vi "ActionVIOnCompile.vi"(8 "error in (no error)":errorcluster, 11 "Device Item Ref in":T1 format="%.0x") -> (0 "error out":errorcluster)   [LabVIEW 2023, in "Vires VTD System Explorer.lvlib"]
uses:
  Vires VTD System Explorer.lvlib
  <vilib>/NI VeriStand/Custom Device API/Custom Device Item Ref.ctl
  Shared/Compiled.Settings.ctl
  RDB Data.ctl
  RDB/RDB Object.ctl
  RDB/RDB Player Object.ctl
  Shared/Network Settings.ctl
  Shared/Protocol.ctl
  Shared/SensorInfos.ctl
  Shared/SensorInfo.ctl
  Shared/Sensor Name.ctl
  MM/MM Data.ctl
  MM/MM Objects.ctl
  MM/MM Object.ctl
  Shared/Timedloop Settings.ctl
  Shared/Constants.vi
  <vilib>/NI VeriStand/Custom Device Tools/Custom Device Utility Library/NI VeriStand - Search for Item by Name.vi
  <vilib>/NI VeriStand/Custom Device API/Get Item Property (Variant).vi
  <vilib>/NI VeriStand/Custom Device API/Set Item Property (Variant).vi
  <vilib>/NI VeriStand/Custom Device API/Custom Device API.lvlib
  <vilib>/NI VeriStand/Custom Device Tools/Custom Device Utility Library/Custom Device Utility Library.lvlib
  <vilib>/NI/NIVS Inline Async API/_Data Access System Explorer/Data Access System Explorer.lvlib
  Shared/Vires VTD Shared.lvlib
  RDB/RDB.lvlib
  MM/MM.lvlib
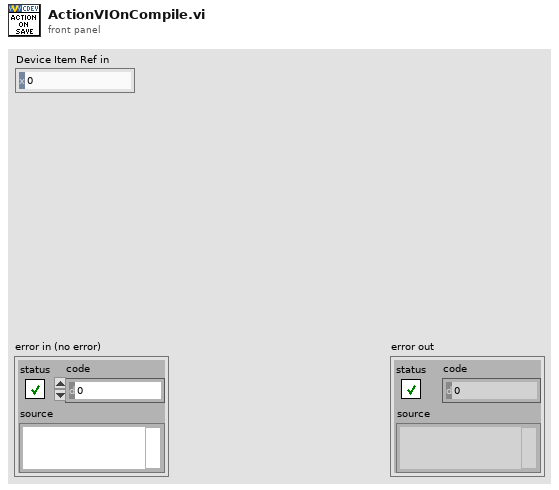
[diagram p1: front panel]
types:
  T1 = typedef "Custom Device API.lvlib/Custom Device Item Ref.ctl" = u64
  T2 = cluster{"Name":string, "Type":enum16{"Output/Write", "Input/Read", "Input/ReadWrite"}, "VS Refs":T1[]}
  T3 = enum16{"Output/Write", "Input/Read", "Input/ReadWrite"}
  T4 = typedef "Vires VTD Shared.lvlib/Compiled.Settings.ctl" = cluster{"Name":string, "RDB Data Receive ":T5, "RDB Data Sent":T5, "vclient":path, "Network Settings":T8, "SensorInfos":T10, "mmanager":path, "Scenario Paths":string[], "Custom SCP Commands":string[], "Timed Loop Settings for TaskControl":T16, "Timed Loop Settings for ModuleManager":T16}
  T5 = typedef "Vires VTD Shared.lvlib/RDB Data.ctl" = T6[]
  T6 = typedef "RDB.lvlib/RDB Object.ctl" = cluster{"pkID":i32, "RDB Player Objects":T7[]}
  T7 = typedef "RDB.lvlib/RDB Player Object.ctl" = cluster{"PlayerID":i32, "Signals":string[], "adv para":i32}
  T8 = typedef "Vires VTD Shared.lvlib/Network Settings.ctl" = cluster{"IP adress":string, "RDB":cluster{"Protocol":T9, "Tx Port":u16, "Rx Port":u16, "Buffer Size":i32, "Timeout":u16}, "SCP":cluster{"Protocol":T9, "Tx Port":u16, "Rx Port":u16, "Buffer Size":i32, "Timeout":u16}}
  T9 = typedef "Vires VTD Shared.lvlib/Protocol.ctl" = enum16{"UDP", "TCP"}
  T10 = typedef "Vires VTD Shared.lvlib/SensorInfos.ctl" = T11[]
  T11 = typedef "Vires VTD Shared.lvlib/SensorInfo.ctl" = cluster{"Sensor Name":T12, "Protocol":T9, "Network port":i32, "# Culled Objects":i32, "PlayerID":u8, "MM Data":T13}
  T12 = typedef "Vires VTD Shared.lvlib/Sensor Name.ctl" = string
  T13 = typedef "Vires VTD Shared.lvlib/MM Data.ctl" = T14[]
  T14 = typedef "MM.lvlib/MM Objects.ctl" = cluster{"pkID":i32, "MM Objects":T15[]}
  T15 = typedef "MM.lvlib/MM Object.ctl" = cluster{"Object":i32, "Signals":string[]}
  T16 = typedef "Vires VTD Shared.lvlib/Timedloop Settings.ctl" = cluster{"Period(ms)":i64, "Priority":i32, "Processor":i32}
  T17 = typedef "Custom Device API.lvlib/Custom Device Item Info.ctl" = cluster{"Name":string, "Is Channel":bool, "GUID":string, "Is Waveform":bool}
  T18 = cluster{"Name":string, "Type":enum16{"Output/Write", "Input/Read", "Input/ReadWrite"}, "VS Refs":T1[]}[]
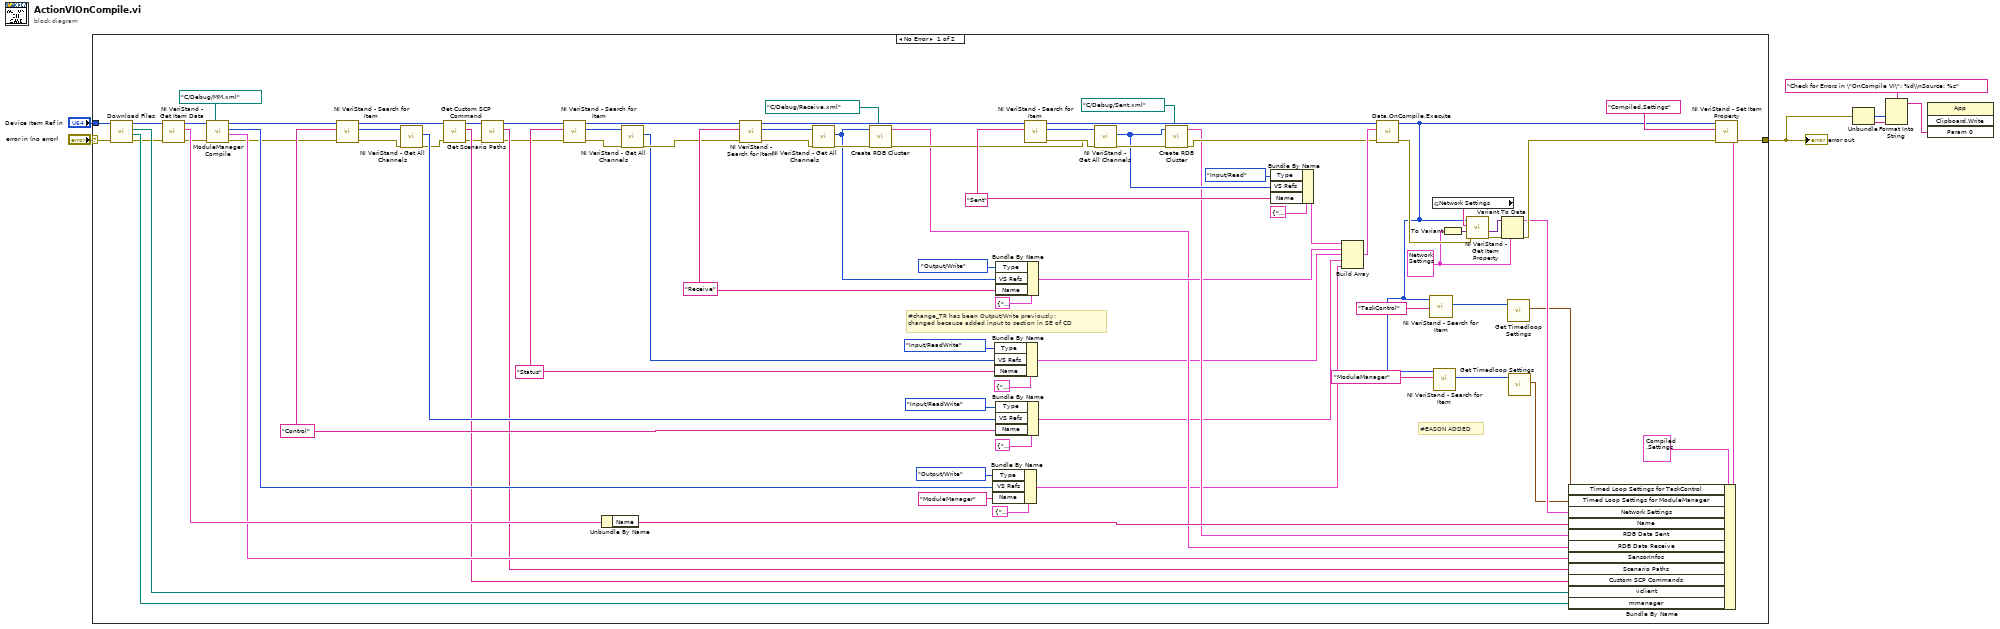
[diagram p0: block diagram]
diagram:
  n1 = case shown="No Error" "error in (no error)" {
    selector: "error in (no error)" -> [w64 w95]
    tunnel: [w66 w95] -> w3
    tunnel: "Device Item Ref in" -> [w65 _]
    frame No Error {
      w30 = "Control" ("Item Name")
      w51 = "Status" ("Item Name")
      w40 = T8 {"IP adress"="127.0.0.1", "RDB"={"Protocol"=enum."UDP", "Tx Port"=48190, "Rx Port"=8192, "Buffer Size"=48190, "Timeout"=10}, "SCP"={"Protocol"=enum."UDP", "Tx Port"=48190, "Rx Port"=8192, "Buffer Size"=48190, "Timeout"=10}} ("UDP Settings")
      w89 = "Sent" ("Item Name")
      w90 = "Receive" ("Item Name")
      # "#EASON ADDED"
      # "#change_TR has been Output/Write previously;\nchanged because added input to section in SE of CD"
      n2 = call "Download Files.vi"("error in (no error)"=w64, "Item Ref in"=w65) -> ("error out"=w20:errorcluster, "mmanager"=w41:path, "vclient"=w43:path, "Device Ref out"=w63:T1)  [unwired: 6 in]
      n3 = call <vilib>:"NI VeriStand - Get Item Data.vi"("error in (no error)"=w20, "Item Ref in"=w63) -> ("error out"=w48:errorcluster, "Item Info"=w92:T17, "Item Ref out"=w49:T1)  [unwired: 6 in, 1 out]
      n4 = call "ModuleManager Compile.vi"("datalog path"=path "C:/Debug/MM.xml", "error in"=w48, "Section Ref in"=w49) -> ("error out"=w28:errorcluster, "SensorInfos"=w42:T10, "Channel Refs"=w45:T1[], "Section Ref out"=w31:T1)  [unwired: 5 in]
      n5 = call-poly <vilib>:"NI VeriStand - Search for Item.vi"("error in"=w28, "Item Name"=w30, "Section Ref in"=w31) -> ("error out"=w33:errorcluster, "Item Ref"=w32:T1, "Section Ref out"=w24:T1)  [unwired: 5 in, 1 out]
      n6 = call <vilib>:"NI VeriStand - Get All Channels.vi"("error in"=w33, "Section Ref in"=w32) -> ("error out"=w27:errorcluster, "Channel Refs"=w29:T1[])  [unwired: 6 in, 2 out]
      n7 = call "Get Custom SCP Command.vi"("error in (no error)"=w27, "Section Ref in"=w24) -> ("error out"=w18:errorcluster, "Custom SCP Commands (str)"=w22:string[], "Section Ref out"=w23:T1)  [unwired: 7 in]
      n8 = call "Get Scenario Paths.vi"("error in (no error)"=w18, "Section Ref in"=w23) -> ("error out"=w19:errorcluster, "Scenario Paths (str)"=w21:string[], "Section Ref out"=w26:T1)  [unwired: 6 in, 1 out]
      n9 = call-poly <vilib>:"NI VeriStand - Search for Item.vi"("error in"=w19, "Item Name"=w51, "Section Ref in"=w26) -> ("error out"=w57:errorcluster, "Item Ref"=w58:T1, "Section Ref out"=w56:T1)  [unwired: 5 in, 1 out]
      n10 = Unbundle By Name(w92) -> ("Name"=w91:string)
      n11 = call <vilib>:"NI VeriStand - Get All Channels.vi"("error in"=w57, "Section Ref in"=w58) -> ("error out"=w55:errorcluster, "Channel Refs"=w52:T1[])  [unwired: 6 in, 2 out]
      n12 = call-poly <vilib>:"NI VeriStand - Search for Item.vi"("error in"=w55, "Item Name"=w90, "Section Ref in"=w56) -> ("error out"=w79:errorcluster, "Item Ref"=w78:T1, "Section Ref out"=w81:T1)  [unwired: 5 in, 1 out]
      n13 = call <vilib>:"NI VeriStand - Get All Channels.vi"("error in"=w79, "Section Ref in"=w78) -> ("error out"=w75:errorcluster, "Channel Refs"=w74:T1[])  [unwired: 6 in, 2 out]
      n14 = call "Create RDB Cluster.vi"("datalog path"=path "C:/Debug/Receive.xml", "error out"=w75, "Channel Refs"=w74) -> ("error out"=w73:errorcluster, "RDB Object"=w67:T5)  [unwired: 7 in]
      n15 = Bundle By Name(cluster=T2 {"Name"="", "Type"=enum."Output/Write", "VS Refs"=[]} ("Group"), "Type"=T3."Output/Write", "VS Refs"=w45, "Name"="ModuleManager") -> (w37:T2)
      n16 = Bundle By Name(cluster=T2 {"Name"="", "Type"=enum."Output/Write", "VS Refs"=[]} ("Group"), "Type"=T3."Input/ReadWrite", "VS Refs"=w52, "Name"=w51) -> (w50:T2)
      n17 = Bundle By Name(cluster=T2 {"Name"="", "Type"=enum."Output/Write", "VS Refs"=[]} ("Group"), "Type"=T3."Output/Write", "VS Refs"=w74, "Name"=w90) -> (w68:T2)
      n18 = Bundle By Name(cluster=T2 {"Name"="", "Type"=enum."Output/Write", "VS Refs"=[]} ("Group"), "Type"=T3."Input/ReadWrite", "VS Refs"=w29, "Name"=w30) -> (w34:T2)
      n19 = call-poly <vilib>:"NI VeriStand - Search for Item.vi"("error in"=w73, "Item Name"=w89, "Section Ref in"=w81) -> ("error out"=w77:errorcluster, "Item Ref"=w76:T1, "Section Ref out"=w82:T1)  [unwired: 5 in, 1 out]
      n20 = call <vilib>:"NI VeriStand - Get All Channels.vi"("error in"=w77, "Section Ref in"=w76) -> ("error out"=w72:errorcluster, "Channel Refs"=w71:T1[])  [unwired: 6 in, 2 out]
      n21 = call "Create RDB Cluster.vi"("datalog path"=path "C:/Debug/Sent.xml", "error out"=w72, "Channel Refs"=w71) -> ("error out"=w70:errorcluster, "RDB Object"=w69:T5)  [unwired: 7 in]
      n22 = Bundle By Name(cluster=T2 {"Name"="", "Type"=enum."Output/Write", "VS Refs"=[]} ("Group"), "Type"=T3."Input/Read", "VS Refs"=w71, "Name"=w89) -> (w87:T2)
      n23 = Build Array(w87, w68, w50, w34, w37) -> (w85:T18)
      n24 = call <vilib>:"Data.OnCompile.Execute.vi"("error in"=w70, "VS Ref Groups"=w85, "Custom Device Ref"=w82) -> ("error out"=w59:errorcluster, "Custom Device Ref"=w17:T1)  [unwired: 7 in]
      n25 = call-poly <vilib>:"NI VeriStand - Search for Item.vi"("Item Name"="TaskControl", "Section Ref in"=w17) -> ("Item Ref"=w16:T1)  [unwired: 6 in, 3 out]
      n26 = global read "Constants.vi" "Network Settings"() -> (w62:string)
      n27 = call-poly <vilib>:"NI VeriStand - Search for Item.vi"("Item Name"="ModuleManager", "Section Ref in"=w17) -> ("Item Ref"=w15:T1)  [unwired: 6 in, 3 out]
      n28 = To Variant(anything=w40) -> (Variant=w39:variant)
      n29 = call-poly <vilib>:"NI VeriStand - Get Item Property.vi"("error in (no error)"=w59, "Default Value"=w39, "Property Name"=w62, "Item Ref in"=w17) -> ("error out"=w61:errorcluster, "Value"=w60:variant)  [unwired: 4 in, 2 out]
      n30 = Variant To Data(error in=w61, type=w40, Variant=w60) -> (data=w25:T8, error out=w38:errorcluster)
      n31 = call "Get Timedloop Settings.vi"("Item Ref in"=w16) -> ("Timed Loop Settings"=w11:T16)  [unwired: 8 in, 2 out]
      n32 = call "Get Timedloop Settings.vi"("Item Ref in"=w15) -> ("Timed Loop Settings"=w12:T16)  [unwired: 8 in, 2 out]
      n33 = Bundle By Name(cluster=T4 {"Name"="", "RDB Data Receive "=[], "RDB Data Sent"=[], "vclient"=path "", "Network Settings"={"IP adress"="127.0.0.1", "RDB"={"Protocol"=enum."UDP", "Tx Port"=48190, "Rx Port"=10, "Buffer Size"=204800, "Timeout"=10}, "SCP"={"Protocol"=enum."TCP", "Tx Port"=48191, "Rx Port"=48191, "Buffer Size"=204800, "Timeout"=10}}, "SensorInfos"=[], "mmanager"=path "", "Scenario Paths"=[], "Custom SCP Commands"=[], "Timed Loop Settings for TaskControl"={"Period(ms)"=2, "Priority"=100, "Processor"=-2}, "Timed Loop Settings for ModuleManager"={"Period(ms)"=2, "Priority"=100, "Processor"=-2}} ("Compiled.Settings"), "Timed Loop Settings for TaskControl"=w11, "Timed Loop Settings for ModuleManager"=w12, "Network Settings"=w25, "Name"=w91, "RDB Data Sent"=w69, "RDB Data Receive"=w67, "SensorInfos"=w42, "Scenario Paths"=w21, "Custom SCP Commands"=w22, "vclient"=w43, "mmanager"=w41) -> (w93:T4)
      n34 = call-poly <vilib>:"NI VeriStand - Set Item Property.vi"("error in (no error)"=w38, "Value"=w93, "Property Name"="Compiled.Settings", "Item Ref in"=w17) -> ("error out"=w66:errorcluster)  [unwired: 5 in, 2 out]
    }
    frame Error {
    }
  }
  "error out" <- w3
  n35 = Unbundle(w3) -> ("code"=w4:i32, "source"=w5:string)  [unwired: 1 out]
  n36 = Format Into String(format string="Check for Errors in \"OnCompile VI\": %d\\nSource: %s", w4, w5) -> (resulting string=w2:string)  [unwired: 2 in, 1 out]
  n37 = invoke class="App" method="Clipboard.Write"("Param 0"=w2) -> ()  [unwired: 3 in, 4 out]
